vi "Publish Actuator Data.vi"(8 "error in (no error)":errorcluster, 11 "Model in":refnum<class "Model.lvclass">) -> (0 "error out":errorcluster, 3 "Model out":refnum<class "Model.lvclass">)   [LabVIEW 2016, in "Model.lvclass"]
uses:
  Model.lvclass
  Model.lvclass/Model.ctl
  User Events/User Events.lvclass/User Events.ctl
  User Events/User Events.lvclass
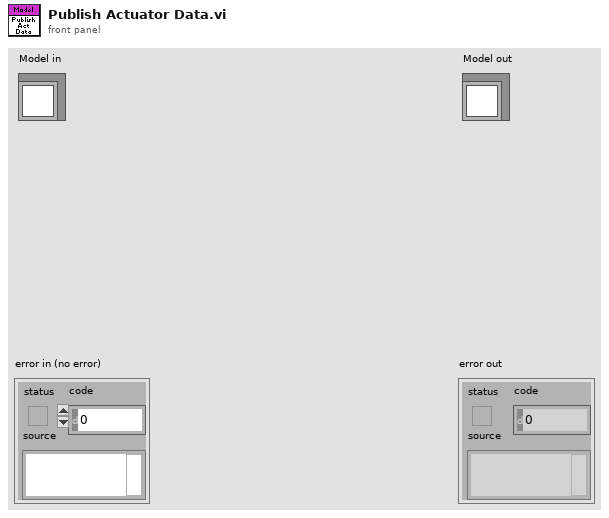
[diagram p1: front panel]
types:
  T1 = typedef "HPMT_Typedefs.lvlib/ActuatorData.ctl" = cluster{"Timestamp":dbl, "Force":dbl, "Encoder Value":i32, "Displacement Sensor 1":dbl, "Displacement Sensor 2":dbl, "Limit Switch CW":bool, "Limit Switch CCW":bool, "Steps Commanded":i32}
  T2 = typedef "HPMT_Typedefs.lvlib/Publish Data Events.ctl" = cluster{"State":refnum<user-event>, "ErrorCode":refnum<user-event>, "Scan Progress":refnum<user-event>, "All Test Status":refnum<user-event>, "ActuatorData":refnum<user-event>, "Test Settings":refnum<user-event>, "Stop Constant Query":refnum<user-event>}
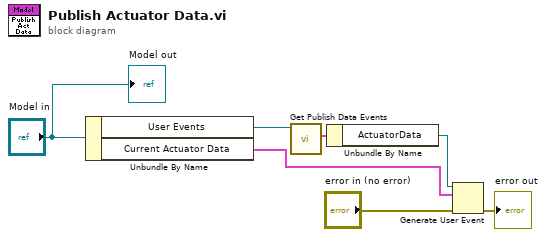
[diagram p0: block diagram]
diagram:
  n1 = Unbundle By Name("Model in") -> ("User Events"=w2:refnum<class "User Events.lvclass">, "Current Actuator Data"=w1:T1)
  n2 = call "Get Publish Data Events.vi"("UserEvents in"=w2) -> ("Publish Data Events"=w6:T2)  [unwired: 9 in, 1 out]
  n3 = Unbundle By Name(w6) -> ("ActuatorData"=w7:refnum<user-event>)
  n4 = Generate User Event(user event=w7, event data cluster=w1, error in="error in (no error)") -> (error out=→"error out":errorcluster)  [unwired: 1 in, 1 out]
  "Model out" <- "Model in"
